vi "Main_Endgame.vi"() -> ()   [LabVIEW 2018]
uses:
  <vilib>/userdefined/High Color/IMAQdx.ctl
  <vilib>/Platform/TimedLoop/XDataNode/timing_clust.ctl
  <vilib>/Platform/TimedLoop/XDataNode/nitl_modes.ctl
  <vilib>/Platform/TimedLoop/XDataNode/wakeup.ctl
  <vilib>/Utility/inputDevices.llb/keyboardAcquire.vi
  <vilib>/Utility/inputDevices.llb/mouseAcquire.vi
  <vilib>/Utility/inputDevices.llb/closeMouse.vi
  <vilib>/Utility/cursorutil.llb/Set Cursor (Icon Pict).vi
  <vilib>/Utility/cursorutil.llb/Set Cursor (Cursor ID).vi
  <vilib>/Platform/TimedLoop/XDataNode/XDataNode.xnode
  <vilib>/Platform/TimedLoop/XDataNode/XDNodeRunTimeDep.lvlib
  <vilib>/vision/driver/NI_Vision_Acquisition_Software.lvlib
panel:
  out "Stop":bool
  in  "default_depth":dbl=120.0
  in  "camera enable":bool
  in  "server port":u16=60006
  in  "listening port":u16=50005
  out "output":dbl[](array[numeric])
  out "beta":dbl
  out "alpha":dbl
  in  "angle_beta_max":dbl=0.2
  in  "angle_beta_min":dbl=-0.7
  in  "angle_alpha_lim":dbl=0.5
  in  "control_region_lim_y":i32=470
  in  "control_region_lim_x":i32=722
  in  "stop_region_lim":i32=90
  in  "UDP enable":bool=TRUE
  in  "Dwell time":dbl=13.0 min=7.0 max=42.0 step=1.0
  out "Boolean 4":bool
  out "Boolean 3":bool
  out "Boolean 2":bool
  out "Boolean":bool
  in  "Cancel Button":bool
  out "Pause_stop":bool
  out "initialized array":i32[](array[numeric])
  out "keys pressed":T1(array[ring])
  out "Local View 2":bool
  out "Image":T2(plugin-control)
  out "Focus":bool
  out "Local View":bool
  out "sd":dbl(graph)
  out "y":i32
  out "x":i32
  out "Global View":bool
  in  "server IP address":string="172.22.11.2"
  out "received data":dbl[](array[numeric])=[0.0, 0.0, 0.0, 0.0, 6000.0]
  out "send data":dbl[](array[numeric])
  out "x_mean":dbl format="%0.2f"
  out "y_mean":dbl format="%0.2f"
  out "y_sd":dbl format="%0.2f"
  out "x_sd":dbl format="%0.2f"
  in  "Stop Button":bool
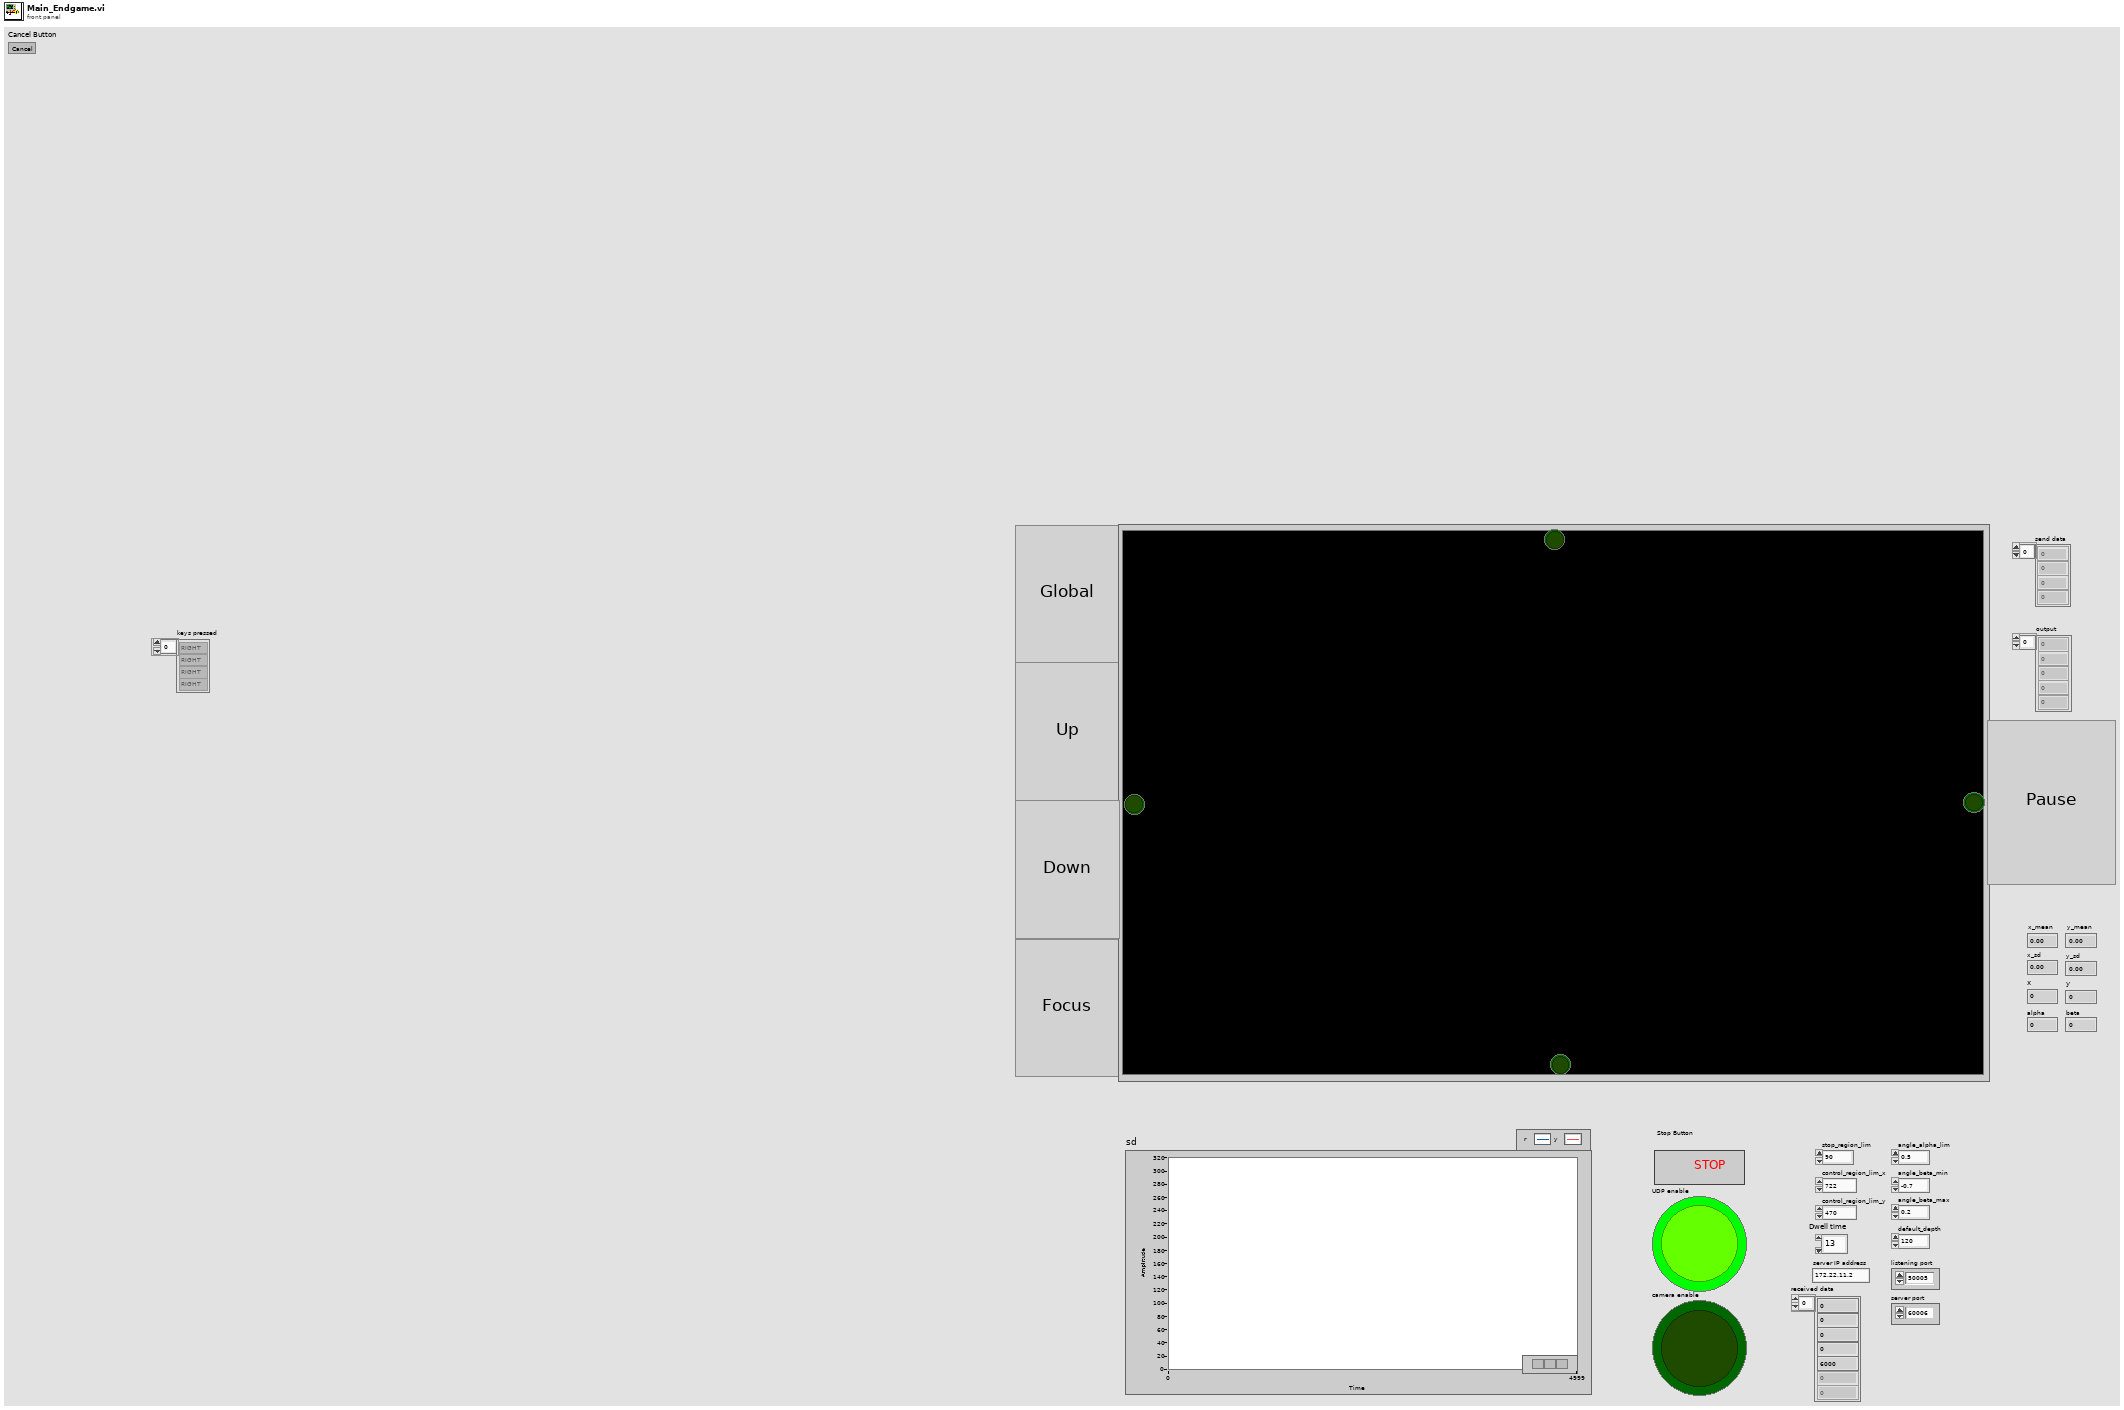
[diagram p1: front panel]
types:
  T1 = enum16{"0", "1", "2", "3", "4", "5", "6", "7", "8", "9", "A", "B", "C", "D", "E", "F", "G", "H", "I", "J", "K", "L", "M", "N", "O", "P", "Q", "R", "S", "T", "U", "V", "W", "X", "Y", "Z", "F1", "F2", "F3", "F4", "F5", "F6", "F7", "F8", "F9", "F10", "F11", "F12", "F13", "F14", "F15", "ADD", "BACK", "BACKSLASH", "CAPITAL", "COMMA", "DECIMAL", "DELETE", "DIVIDE", "DOWN", "END", "EQUALS", "ESCAPE", "GRAVE (`)", "HOME", "INSERT", "LBRACKET", "LCONTROL", "LEFT", "L ALT", "LSHIFT", "LWIN", "MINUS", "MULTIPLY", "NEXT", "NUMLOCK", "NUMPAD_0", "NUMPAD_1", "NUMPAD_2", "NUMPAD_3", "NUMPAD_4", "NUMPAD_5", "NUMPAD_6", "NUMPAD_7", "NUMPAD_8", "NUMPAD_9", "PAUSE", "PERIOD", "PRIOR (PG UP)", "RBRACKET", "RCONTROL", "RETURN", "RIGHT", "R ALT", "RSHIFT", "RWIN", "SCROLL", "SEMICOLON", "SLASH", "SPACE", "SUBTRACT", "TAB", "UP", "ENTER (num pad)", "' (quote)"}[]
  T2 = typedef "IMAQ Image.ctl" = refnum<image>
  T3 = enum16{"0", "1", "2", "3", "4", "5", "6", "7", "8", "9", "A", "B", "C", "D", "E", "F", "G", "H", "I", "J", "K", "L", "M", "N", "O", "P", "Q", "R", "S", "T", "U", "V", "W", "X", "Y", "Z", "F1", "F2", "F3", "F4", "F5", "F6", "F7", "F8", "F9", "F10", "F11", "F12", "F13", "F14", "F15", "ADD", "BACK", "BACKSLASH", "CAPITAL", "COMMA", "DECIMAL", "DELETE", "DIVIDE", "DOWN", "END", "EQUALS", "ESCAPE", "GRAVE (`)", "HOME", "INSERT", "LBRACKET", "LCONTROL", "LEFT", "L ALT", "LSHIFT", "LWIN", "MINUS", "MULTIPLY", "NEXT", "NUMLOCK", "NUMPAD_0", "NUMPAD_1", "NUMPAD_2", "NUMPAD_3", "NUMPAD_4", "NUMPAD_5", "NUMPAD_6", "NUMPAD_7", "NUMPAD_8", "NUMPAD_9", "PAUSE", "PERIOD", "PRIOR (PG UP)", "RBRACKET", "RCONTROL", "RETURN", "RIGHT", "R ALT", "RSHIFT", "RWIN", "SCROLL", "SEMICOLON", "SLASH", "SPACE", "SUBTRACT", "TAB", "UP", "ENTER (num pad)", "' (quote)"}
  T4 = typedef "XDNodeRunTimeDep.lvlib/timing_clust.ctl" = cluster{"Expected End [f-1]":u64, "Actual End [f-1]":u64, "Finished Late? [f-1]":bool, "Expected End [i-1]":u64, "Actual End [i-1]":u64, "Finished Late? [i-1]":bool, "Expected Start [i]":u64, "Actual Start [i]":u64, "Expected Start [f]":u64, "Actual Start [f]":u64, "Source Name":string, "Structure Name":string, "Period":i64, "Deadline":i64, "Offset":i64, "Start":i64, "Priority":i32, "Timeout":i32, "Mode":T5, "Wakeup Reason":T6, "Error":errorcluster, "Source Type":string, "Secondary Source Type":string, "Global End Time":u64, "Global Start Time":u64, "Frame Duration":u64, "Iteration Duration":u64, "Assigned CPU":i32, "I/O Scan Engine Mode":u32}
  T5 = typedef "XDNodeRunTimeDep.lvlib/nitl_modes.ctl" = enum32{"No Change", "Process missed periods, maintain original phase", "Discard missed periods, maintain original phase", "Process missed periods, ignore original phase", "Discard missed periods, ignore original phase"}
  T6 = typedef "XDNodeRunTimeDep.lvlib/wakeup.ctl" = enum32{"Normal", "Aborted", "Asynchronous wakeup", "Timing source error", "Timed loop error", "Timeout"}
  T7 = typedef "LVRectTypeDef.ctl" = cluster{"Left":i16, "Top":i16, "Right":i16, "Bottom":i16}
  T8 = cluster{"Horizontal":i32, "Vertical":i32, "Scrolling":i32}
  T9 = typedef "LVPointTypeDef.ctl" = cluster{"Horizontal":i16, "Vertical":i16}
  T10 = typedef "IMAQdx.ctl" = refnum<k21>
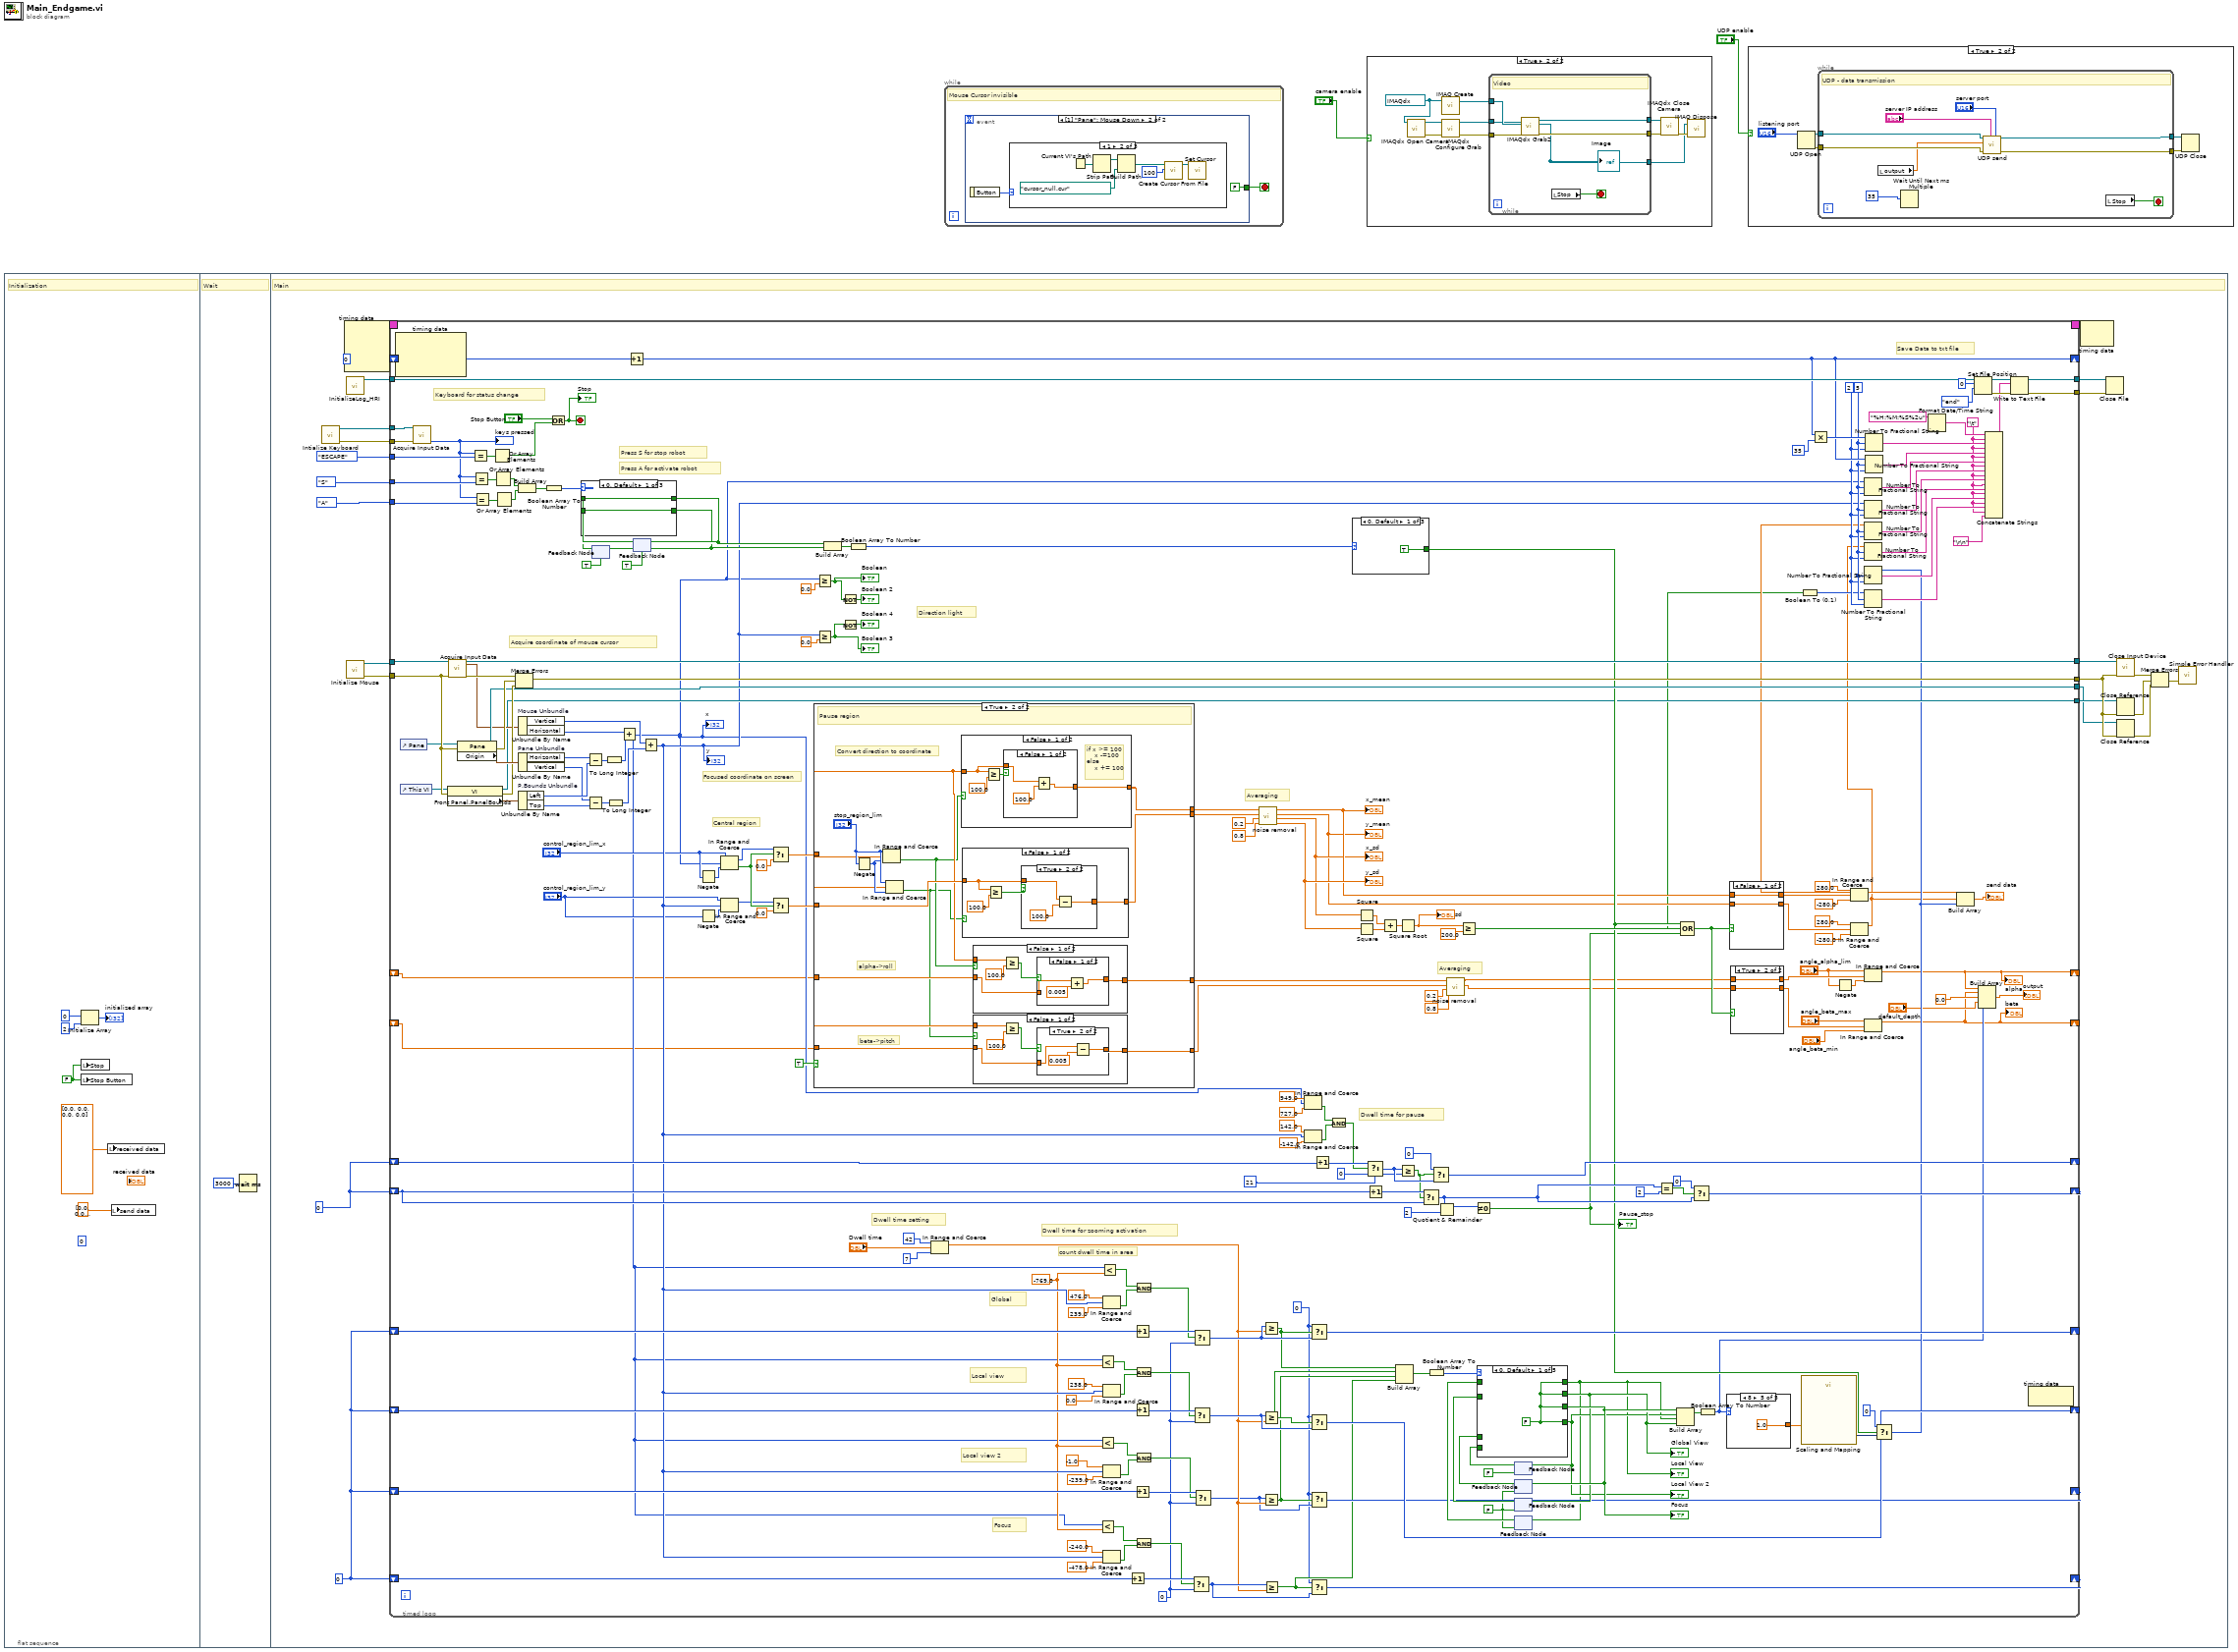
[diagram p0: block diagram]
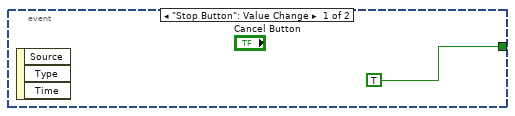
[diagram p4: hidden frame]
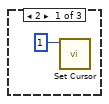
[diagram p5: hidden frame]
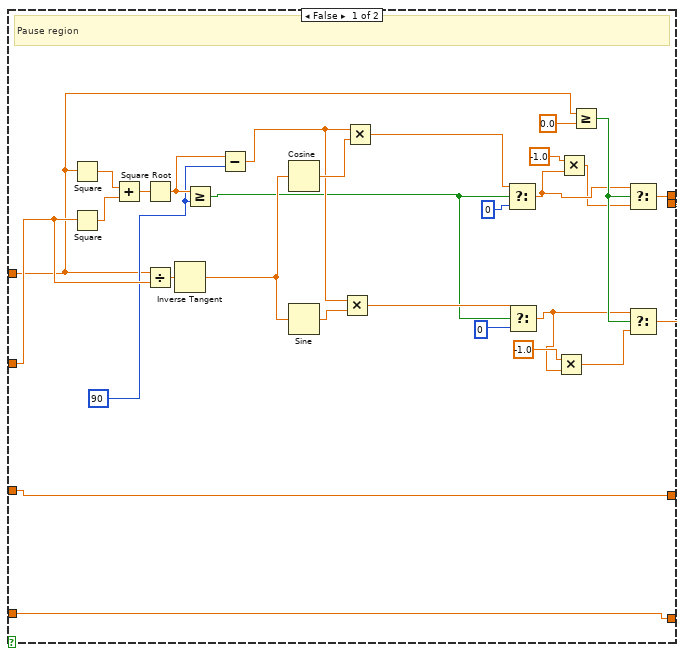
[diagram p8: hidden frame]
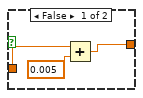
[diagram p9: hidden frame]
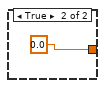
[diagram p10: hidden frame]
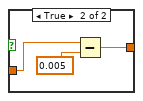
[diagram p11: hidden frame]
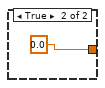
[diagram p12: hidden frame]
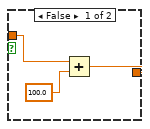
[diagram p13: hidden frame]
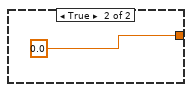
[diagram p14: hidden frame]
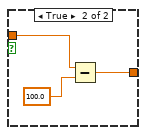
[diagram p15: hidden frame]
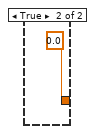
[diagram p16: hidden frame]
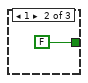
[diagram p17: hidden frame]
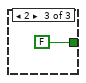
[diagram p18: hidden frame]
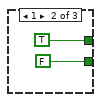
[diagram p19: hidden frame]
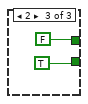
[diagram p20: hidden frame]
diagram:
  n1 = flat-sequence {
    frame #0 {
      (unwired) 0
      w3 = FALSE
      # "Initialization"
      n2 = Initialize Array(0, 2) -> (→"initialized array":i32[])
      n3 = local write "Stop"(w3) -> ()
      n4 = local write "Stop Button"(w3) -> ()
      n5 = local write "received data"(dbl[] [0.0, 0.0, 0.0, 0.0] ("appended array")) -> ()
      n6 = local write "send data"(dbl[] [0.0, 0.0, 0.0, 0.0, 0.0]) -> ()
    }
    frame #1 {
      # "Wait"
      n7 = Wait (ms)(milliseconds to wait=3000) -> ()  [unwired: 1 out]
    }
    frame #2 {
      w12 = 0
      w11 = 0
      # "Main"
      n8 = call <vilib>:"Intialize Keyboard.vi"() -> ("error out"=w19:errorcluster, "device ID"=w20:refnum<k1>)  [unwired: 10 in]
      n9 = node-c288() -> (w32:T4)  [unwired: 4 in]
      n10 = call "InitializeLog_HRI.vi"() -> ("refnum out"=w14:refnum<file>)  [unwired: 11 in]
      n11 = call <vilib>:"Initialize Mouse.vi"() -> ("error out"=w25:errorcluster, "device ID"=w26:refnum<k1>)  [unwired: 10 in]
      n12 = timed-loop {
        timing: w32 -> [_]
        timing-out: [_] -> w31
        shift-right: [w213] -> _
        shift-left: w12 -> [w247]
        shift-right: [w196] -> _
        shift-left: w12 -> [w246]
        tunnel: w26 -> [w232]
        tunnel: w25 -> [w231]
        tunnel: [w228] -> w24
        tunnel: [w227] -> w23
        tunnel: [w226] -> w22
        tunnel: [w116] -> w21
        shift-right: [w215] -> _
        shift-left: w12 -> [w221]
        shift-right: [w194] -> _
        shift-left: w12 -> [w199]
        tunnel: w20 -> [w177]
        tunnel: w19 -> [w176]
        tunnel: T3."ESCAPE" ("keyType 3") -> [w175]
        tunnel: T3."S" ("keyType 3") -> [w174]
        tunnel: T3."A" ("keyType 3") -> [w173]
        tunnel: [w147] -> w15
        tunnel: w14 -> [w146]
        shift-right: [w142] -> _
        shift-left: 0 -> [w145]
        shift-right: [w140] -> _
        shift-left: w11 -> [w141]
        shift-right: [w133] -> _
        shift-left: w11 -> [w138]
        shift-right: [w42] -> _
        shift-left: _ -> [w57]
        shift-right: [w41] -> _
        shift-left: _ -> [w56]
        tunnel: [w47] -> w10
        stop <- w40 stop-if-true
        w118 = 2
        w119 = 5
        w120 = "\t"
        w46 = 0
        w186 = FALSE
        w39 = 0
        w75 = -769.0
        # "count dwell time in area"
        # "Focus"
        # "Local view 2"
        # "Local view"
        # "Global"
        # "Averaging"
        # "Central region"
        # "Focused coordinate on screen"
        # "Averaging"
        # "Keyboard for status change"
        # "Acquire coordinate of mouse cursor"
        # "Direction light"
        # "Dwell time for pause"
        # "Dwell time for zooming activation"
        # "Save Data to txt file"
        # "Dwell time setting"
        # "Press A for activate robot"
        # "Press S for stop robot"
        n13 = node-c288() -> ()  [unwired: 1 in, 4 out]
        n14 = control-ref of="Pane"() -> (w230:refnum<vi>)
        n15 = control-ref of="This VI"() -> (w229:refnum<vi>)
        n16 = call-poly <vilib>:"Acquire Input Data.vi"("device ID"=w177, "error in (no error)"=w176) -> ("keys pressed"=w111:T1)  [unwired: 15 in, 2 out]
        "keys pressed" <- w111
        n17 = property class="VI"(reference=w229, error in=w231) -> (reference out=w116:refnum<vi>, error out=w235:errorcluster, "Front Panel.PanelBounds"=w244:T7)
        n18 = call-poly <vilib>:"Acquire Input Data.vi"("device ID"=w232, "error in (no error)"=w231) -> ("device ID"=w228:refnum<k1>, "axis info"=w225:T8, "error out"=w238:errorcluster)  [unwired: 14 in, 1 out]
        n19 = property class="Pane"(reference=w230, error in=w231) -> (reference out=w226:refnum<vi>, error out=w236:errorcluster, "Origin"=w245:T9)
        n20 = Equal?(x=w111, y=w175) -> (x = y?=w180:bool[])
        n21 = Equal?(x=w111, y=w174) -> (x = y?=w179:bool[])
        n22 = Equal?(x=w111, y=w173) -> (x = y?=w178:bool[])
        n23 = Or Array Elements(Boolean array=w180) -> (logical OR=w104:bool)
        n24 = Or Array Elements(Boolean array=w179) -> (logical OR=w105:bool)
        n25 = Or Array Elements(Boolean array=w178) -> (logical OR=w163:bool)
        n26 = Merge Errors(w238, w236, w235) -> (w227:errorcluster)
        n27 = Unbundle By Name "Mouse Unbundle"(w225) -> ("Vertical"=w224:i32, "Horizontal"=w223:i32)
        n28 = Unbundle By Name "Pane Unbundle"(w245) -> ("Horizontal"=w243:i16, "Vertical"=w241:i16)
        n29 = Unbundle By Name "P.Bounds Unbundle"(w244) -> ("Left"=w242:i16, "Top"=w240:i16)
        n30 = Build Array(w105, w163) -> (w171:bool[])
        n31 = Boolean Array To Number(Boolean array=w171) -> (number=w172:u32)
        n32 = Or(x="Stop Button", y=w104) -> (x .or. y?=w40:bool)
        "Stop" <- w40
        n33 = Subtract(x=w243, y=w242) -> (x-y=w237:i16)
        n34 = Subtract(x=w241, y=w240) -> (x-y=w239:i16)
        n35 = feedback #1(TRUE) -> (w167:bool)
        n36 = To Long Integer(number=w237) -> (32bit integer=w234:i32)
        n37 = To Long Integer(number=w239) -> (32bit integer=w233:i32)
        n38 = Add(x=w223, y=w234) -> (x+y=w60:i32)
        "x" <- w60
        n39 = Increment(x=w145) -> (x+1=w142:i32)
        n40 = feedback #2(TRUE) -> (w168:bool)
        n41 = case shown="0, Default" w172 {
          tunnel: [w356 FALSE TRUE] -> w165
          tunnel: [w357 TRUE FALSE] -> w166
          tunnel: w168 -> [w357 _ _]
          tunnel: w167 -> [w356 _ _]
          frame 0, Default {
          }
          frame 1 {
          }
          frame 2 {
          }
        }
        n42 = feedback-in #1(w165) -> ()
        n43 = feedback-in #2(w166) -> ()
        n44 = Add(x=w224, y=w233) -> (x+y=w79:i32)
        "y" <- w79
        n45 = Negate(x="control_region_lim_x") -> (-x=w64:i32)
        n46 = Negate(x="control_region_lim_y") -> (-x=w62:i32)
        n47 = In Range and Coerce(upper limit="control_region_lim_x", x=w60, lower limit=w64) -> (coerced(x)=w125:i32, In Range?=w126:bool)
        n48 = In Range and Coerce(upper limit="control_region_lim_y", x=w79, lower limit=w62) -> (coerced(x)=w124:i32)  [unwired: 1 out]
        n49 = Select(t=w125, s=w126, f=0.0) -> (s? t:f=w129:dbl)
        n50 = Select(t=w124, s=w126, f=0.0) -> (s? t:f=w127:dbl)
        n51 = case shown="True" TRUE {
          tunnel: w129 -> [w278 w297]
          tunnel: w127 -> [w291 w298]
          tunnel: [w268 w306] -> w107
          tunnel: [w270 w305] -> w106
          tunnel: w57 -> [w267 w302]
          tunnel: [w267 w301] -> w38
          tunnel: w56 -> [w266 w300]
          tunnel: [w266 w299] -> w35
          frame False {
            w287 = 90
            # "Pause region"
            n52 = Square(x=w278) -> (x^2=w292:dbl)
            n53 = Square(x=w291) -> (x^2=w294:dbl)
            n54 = Add(x=w292, y=w294) -> (x+y=w293:dbl)
            n55 = Square Root(x=w293) -> (sqrt(x)=w288:dbl)
            n56 = Divide(x=w278, y=w291) -> (x/y=w286:dbl)
            n57 = Inverse Tangent(1:w286) -> (0:w285:dbl)
            n58 = Greater Or Equal?(x=w288, y=w287) -> (x >= y?=w269:bool)
            n59 = Subtract(x=w288, y=w287) -> (x-y=w281:dbl)
            n60 = Cosine(x=w285) -> (cos(x)=w284:dbl)
            n61 = Sine(x=w285) -> (sin(x)=w282:dbl)
            n62 = Multiply(x=w281, y=w282) -> (x*y=w280:dbl)
            n63 = Multiply(x=w281, y=w284) -> (x*y=w283:dbl)
            n64 = Select(t=w283, s=w269, f=0) -> (s? t:f=w275:dbl)
            n65 = Select(t=w280, s=w269, f=0) -> (s? t:f=w272:dbl)
            n66 = Multiply(x=-1.0, y=w272) -> (x*y=w271:dbl)
            n67 = Multiply(x=-1.0, y=w275) -> (x*y=w274:dbl)
            n68 = Greater Or Equal?(x=w278, y=0.0) -> (x >= y?=w277:bool)
            n69 = Select(t=w275, s=w277, f=w274) -> (s? t:f=w268:dbl)
            n70 = Select(t=w272, s=w277, f=w271) -> (s? t:f=w270:dbl)
          }
          frame True {
            # "beta->pitch"
            # "alpha->roll"
            # "Convert direction to coordinate"
            # "Pause region"
            n71 = Negate(x="stop_region_lim") -> (-x=w303:i32)
            n72 = In Range and Coerce(upper limit="stop_region_lim", x=w297, lower limit=w303) -> (In Range?=w296:bool)  [unwired: 1 out]
            n73 = In Range and Coerce(upper limit="stop_region_lim", x=w298, lower limit=w303) -> (In Range?=w295:bool)  [unwired: 1 out]
            n74 = case shown="False" w296 {
              tunnel: w297 -> [w343 _]
              tunnel: [w342 0.0] -> w306
              frame False {
                # "if x >= 100 \n    x -=100\nelse\n    x += 100"
                n75 = Greater Or Equal?(x=w343, y=100.0) -> (x >= y?=w345:bool)
                n76 = case shown="False" w345 {
                  tunnel: w343 -> [w347 w350]
                  tunnel: [w346 w349] -> w342
                  frame False {
                    n77 = Add(x=w347, y=100.0) -> (x+y=w346:dbl)
                  }
                  frame True {
                    n78 = Subtract(x=w350, y=100.0) -> (x-y=w349:dbl)
                  }
                }
              }
              frame True {
              }
            }
            n79 = case shown="False" w295 {
              tunnel: [w332 0.0] -> w305
              tunnel: w298 -> [w331 _]
              frame False {
                n80 = Greater Or Equal?(x=w331, y=100.0) -> (x >= y?=w334:bool)
                n81 = case shown="True" w334 {
                  tunnel: w331 -> [w336 w339]
                  tunnel: [w335 w338] -> w332
                  frame False {
                    n82 = Add(x=w336, y=100.0) -> (x+y=w335:dbl)
                  }
                  frame True {
                    n83 = Subtract(x=w339, y=100.0) -> (x-y=w338:dbl)
                  }
                }
              }
              frame True {
              }
            }
            n84 = case shown="False" w296 {
              tunnel: w302 -> [w321 _]
              tunnel: [w320 0.0] -> w301
              tunnel: w297 -> [w319 _]
              frame False {
                n85 = Greater Or Equal?(x=w319, y=100.0) -> (x >= y?=w323:bool)
                n86 = case shown="False" w323 {
                  tunnel: w321 -> [w325 w327]
                  tunnel: [w324 w328] -> w320
                  frame False {
                    n87 = Add(x=w325, y=0.005) -> (x+y=w324:dbl)
                  }
                  frame True {
                    n88 = Subtract(x=w327, y=0.005) -> (x-y=w328:dbl)
                  }
                }
              }
              frame True {
              }
            }
            n89 = case shown="False" w295 {
              tunnel: w300 -> [w308 _]
              tunnel: [w309 0.0] -> w299
              tunnel: w298 -> [w307 _]
              frame False {
                n90 = Greater Or Equal?(x=w307, y=100.0) -> (x >= y?=w311:bool)
                n91 = case shown="True" w311 {
                  tunnel: w308 -> [w313 w315]
                  tunnel: [w312 w316] -> w309
                  frame False {
                    n92 = Add(x=w313, y=0.005) -> (x+y=w312:dbl)
                  }
                  frame True {
                    n93 = Subtract(x=w315, y=0.005) -> (x-y=w316:dbl)
                  }
                }
              }
              frame True {
              }
            }
          }
        }
        n94 = Greater Or Equal?(x=w60, y=0.0) -> (x >= y?=w115:bool)
        "Boolean" <- w115
        n95 = Greater Or Equal?(x=w79, y=0.0) -> (x >= y?=w113:bool)
        "Boolean 3" <- w113
        n96 = Build Array(w166, w165) -> (w164:bool[])
        n97 = Not(x=w115) -> (.not. x?=→"Boolean 2":bool)
        n98 = Not(x=w113) -> (.not. x?=→"Boolean 4":bool)
        n99 = Boolean Array To Number(Boolean array=w164) -> (number=w161:u32)
        n100 = In Range and Coerce(upper limit=42, x="Dwell time", lower limit=7) -> (coerced(x)=w103:dbl)  [unwired: 1 out]
        n101 = Less?(x=w60, y=w75) -> (x < y?=w183:bool)
        n102 = Less?(x=w60, y=w75) -> (x < y?=w182:bool)
        n103 = Less?(x=w60, y=w75) -> (x < y?=w181:bool)
        n104 = Less?(x=w60, y=w75) -> (x < y?=w184:bool)
        n105 = In Range and Coerce(upper limit=476.0, x=w79, lower limit=239.0) -> (In Range?=w222:bool)  [unwired: 1 out]
        n106 = In Range and Coerce(upper limit=238.0, x=w79, lower limit=0.0) -> (In Range?=w250:bool)  [unwired: 1 out]
        n107 = In Range and Coerce(upper limit=-1.0, x=w79, lower limit=-239.0) -> (In Range?=w255:bool)  [unwired: 1 out]
        n108 = In Range and Coerce(upper limit=-240.0, x=w79, lower limit=-478.0) -> (In Range?=w202:bool)  [unwired: 1 out]
        n109 = Increment(x=w199) -> (x+1=w204:i32)
        n110 = Increment(x=w221) -> (x+1=w220:i32)
        n111 = Increment(x=w247) -> (x+1=w252:i32)
        n112 = Increment(x=w246) -> (x+1=w257:i32)
        n113 = And(x=w184, y=w222) -> (x .and. y?=w219:bool)
        n114 = And(x=w183, y=w250) -> (x .and. y?=w251:bool)
        n115 = And(x=w182, y=w255) -> (x .and. y?=w256:bool)
        n116 = And(x=w181, y=w202) -> (x .and. y?=w203:bool)
        n117 = Select(t=w204, s=w203, f=w46) -> (s? t:f=w195:i32)
        n118 = Select(t=w220, s=w219, f=w46) -> (s? t:f=w216:i32)
        n119 = Select(t=w252, s=w251, f=w46) -> (s? t:f=w214:i32)
        n120 = Select(t=w257, s=w256, f=w46) -> (s? t:f=w73:i32)
        n121 = call "noise removal.vi"("after14"=0.8, "before14"=0.2, "y"=w106, "x"=w107) -> ("sdy"=w84:dbl, "sdx"=w82:dbl, "newy"=w81:dbl, "newx"=w83:dbl)  [unwired: 4 in]
        "x_mean" <- w83
        "y_mean" <- w81
        "y_sd" <- w84
        "x_sd" <- w82
        n122 = Greater Or Equal?(x=w216, y=w103) -> (x >= y?=w208:bool)
        n123 = Greater Or Equal?(x=w214, y=w103) -> (x >= y?=w74:bool)
        n124 = Greater Or Equal?(x=w73, y=w103) -> (x >= y?=w72:bool)
        n125 = Greater Or Equal?(x=w195, y=w103) -> (x >= y?=w193:bool)
        n126 = In Range and Coerce(upper limit=949.0, x=w60, lower limit=727.0) -> (In Range?=w88:bool)  [unwired: 1 out]
        n127 = In Range and Coerce(upper limit=142.0, x=w79, lower limit=-142.0) -> (In Range?=w100:bool)  [unwired: 1 out]
        n128 = Select(t=w39, s=w208, f=w216) -> (s? t:f=w215:i32)
        n129 = Select(t=w39, s=w74, f=w214) -> (s? t:f=w213:i32)
        n130 = Select(t=w39, s=w72, f=w73) -> (s? t:f=w196:i32)
        n131 = Select(t=w39, s=w193, f=w195) -> (s? t:f=w194:i32)
        n132 = Increment(x=w141) -> (x+1=w99:i32)
        n133 = And(x=w88, y=w100) -> (x .and. y?=w97:bool)
        n134 = case shown="0, Default" w161 {
          tunnel: [TRUE FALSE FALSE] -> w131
          frame 0, Default {
          }
          frame 1 {
          }
          frame 2 {
          }
        }
        n135 = Square(x=w82) -> (x^2=w261:dbl)
        n136 = Square(x=w84) -> (x^2=w260:dbl)
        n137 = Select(t=w99, s=w97, f=0) -> (s? t:f=w95:i32)
        n138 = Increment(x=w138) -> (x+1=w90:i32)
        n139 = Add(x=w261, y=w260) -> (x+y=w259:dbl)
        n140 = Build Array(w208, w74, w72, w193) -> (w218:bool[])
        n141 = Square Root(x=w259) -> (sqrt(x)=w80:dbl)
        "sd" <- w80
        n142 = Greater Or Equal?(x=w95, y=21) -> (x >= y?=w89:bool)
        n143 = Select(t=w90, s=w89, f=w138) -> (s? t:f=w134:i32)
        n144 = Boolean Array To Number(Boolean array=w218) -> (number=w217:u32)
        n145 = Select(t=0, s=w89, f=w95) -> (s? t:f=w140:i32)
        n146 = Quotient & Remainder(x=w134, y=2) -> (x-y*floor(x/y)=w45:i32)  [unwired: 1 out]
        n147 = call "noise removal.vi"("after14"=0.8, "before14"=0.2, "y"=w35, "x"=w38) -> ("newy"=w36:dbl, "newx"=w37:dbl)  [unwired: 4 in, 2 out]
        n148 = Greater Or Equal?(x=w80, y=200.0) -> (x >= y?=w139:bool)
        n149 = Not Equal To 0?(x=w45) -> (x != 0?=w44:bool)
        "Pause_stop" <- w44
        n150 = feedback #3(FALSE) -> (w210:bool)
        n151 = feedback #4(w186) -> (w211:bool)
        n152 = feedback #5(w186) -> (w207:bool)
        n153 = feedback #6(w186) -> (w198:bool)
        n154 = case shown="0, Default" w217 {
          tunnel: [w367 TRUE FALSE w377 w379] -> w205
          tunnel: w211 -> [_ _ _ _ _]
          tunnel: [w367 FALSE TRUE w377 w379] -> w192
          tunnel: w210 -> [_ _ _ _ _]
          tunnel: [w367 FALSE FALSE FALSE TRUE] -> w197
          tunnel: w207 -> [_ _ _ _ _]
          tunnel: [w367 FALSE FALSE TRUE w379] -> w191
          tunnel: w198 -> [_ _ _ _ _]
          frame 0, Default {
            w367 = FALSE
          }
          frame 1 {
          }
          frame 2 {
          }
          frame 4 {
            w377 = FALSE
          }
          frame 8 {
            w379 = FALSE
          }
        }
        "Global View" <- w197
        "Local View" <- w191
        "Focus" <- w205
        "Local View 2" <- w192
        n155 = feedback-in #3(w192) -> ()
        n156 = feedback-in #4(w205) -> ()
        n157 = feedback-in #5(w197) -> ()
        n158 = feedback-in #6(w191) -> ()
        n159 = Equal?(x=w134, y=2) -> (x = y?=w136:bool)
        n160 = Build Array(w205, w192, w191, w197) -> (w209:bool[])
        n161 = Compound Arithmetic op=OR(w131, w139, w44) -> (w43:bool)
        n162 = Select(t=0, s=w136, f=w134) -> (s? t:f=w133:i32)
        n163 = Boolean Array To Number(Boolean array=w209) -> (number=w48:u32)
        n164 = case shown="8" w48 {
          tunnel: [1.0 1.8 1.5 1.2 1.0] -> w206
          frame 0, Default {
          }
          frame 1 {
          }
          frame 2 {
          }
          frame 4 {
          }
          frame 8 {
          }
        }
        n165 = case shown="False" w43 {
          tunnel: [w382 w383] -> w102
          tunnel: [w381 w383] -> w101
          tunnel: w83 -> [w382 _]
          tunnel: w81 -> [w381 _]
          frame False {
          }
          frame True {
            w383 = 0.0
          }
        }
        n166 = case shown="True" w43 {
          tunnel: [w263 w265] -> w59
          tunnel: [w262 w264] -> w58
          tunnel: w37 -> [w263 w265]
          tunnel: w36 -> [w262 w264]
          frame False {
          }
          frame True {
          }
        }
        n167 = Boolean To (0,1)(Boolean=w43) -> (0, 1=w117:i16)
        n168 = call "Scaling and Mapping"("Signals"=w206) -> ("Scaled Signals"=w160:dynamicdata)  [unwired: 9 in, 1 out]
        n169 = Multiply(x=w142, y=35) -> (x*y=w143:i32)
        n170 = Negate(x="angle_alpha_lim") -> (-x=w55:dbl)
        n171 = In Range and Coerce(upper limit=280.0, x=w102, lower limit=-280.0) -> (coerced(x)=w70:dbl)  [unwired: 1 out]
        n172 = In Range and Coerce(upper limit=280.0, x=w101, lower limit=-280.0) -> (coerced(x)=w69:dbl)  [unwired: 1 out]
        n173 = Number To Fractional String(number=w69, width (-)=w119, precision (6)=w118) -> (F-format string=w123:string)  [unwired: 1 in]
        n174 = In Range and Coerce(upper limit="angle_alpha_lim", x=w59, lower limit=w55) -> (coerced(x)=w42:dbl)  [unwired: 1 out]
        "alpha" <- w42
        n175 = In Range and Coerce(upper limit="angle_beta_max", x=w58, lower limit="angle_beta_min") -> (coerced(x)=w41:dbl)  [unwired: 1 out]
        "beta" <- w41
        n176 = Number To Fractional String(number=w60, width (-)=w119, precision (6)=w118) -> (F-format string=w156:string)  [unwired: 1 in]
        n177 = Number To Fractional String(number=w79, width (-)=w119, precision (6)=w118) -> (F-format string=w149:string)  [unwired: 1 in]
        n178 = Number To Fractional String(number=w70, width (-)=w119, precision (6)=w118) -> (F-format string=w148:string)  [unwired: 1 in]
        n179 = Number To Fractional String(number=w117, width (-)=w119, precision (6)=w118) -> (F-format string=w121:string)  [unwired: 1 in]
        n180 = Number To Fractional String(number=w143, width (-)=w119, precision (6)=w118) -> (F-format string=w158:string)  [unwired: 1 in]
        n181 = Number To Fractional String(number=w142, width (-)=w119, precision (6)=w118) -> (F-format string=w157:string)  [unwired: 1 in]
        n182 = Select(t=0, s=w131, f=w160) -> (s? t:f=w71:i32)
        n183 = Number To Fractional String(number=w71, width (-)=w119, precision (6)=w118) -> (F-format string=w122:string)  [unwired: 1 in]
        n184 = Format Date/Time String(time format string (%c)="%H:%M:%S%2u") -> (date/time string=w150:string)  [unwired: 2 in]
        n185 = Build Array(w70, w69, w71) -> (→"send data":dbl[])
        n186 = Set File Position(offset (in bytes) (0)=i64 0, refnum=w146, from (0:start)=enum16{"start", "end", "current"}."end") -> (refnum out=w153:refnum<file>, error out=w159:errorcluster)  [unwired: 1 in]
        n187 = Build Array(w42, w41, 0.0, "default_depth", w48) -> (→"output":dbl[])
        n188 = Concatenate Strings(w150, w120, w158, w120, w157, w120, w156, w120, w149, w120, w148, w120, w123, w120, w122, w120, w121, w120, "\r\n") -> (w152:string)
        n189 = Write to Text File(file (use dialog)=w153, text=w152, error in=w159) -> (refnum out=w147:refnum<file>, error out=w47:errorcluster)  [unwired: 1 in, 1 out]
        n190 = node-c288() -> ()  [unwired: 1 in, 1 out]
      }
      n191 = node-c288(w31) -> ()  [unwired: 1 out]
      n192 = Close File(refnum=w15, error in=w10) -> ()  [unwired: 2 out]
      n193 = call-poly <vilib>:"Close Input Device.vi"("error in (no error)"=w23, "device ID"=w24) -> ("error out"=w30:errorcluster)  [unwired: 8 in]
      n194 = Close Reference(reference=w22, error in (no error)=w23) -> (error out=w29:errorcluster)
      n195 = Close Reference(reference=w21, error in (no error)=w23) -> (error out=w28:errorcluster)
      n196 = Merge Errors(w30, w29, w28) -> (w27:errorcluster)
      n197 = call <vilib>:"Simple Error Handler.vi"("error in (no error)"=w27) -> ()  [unwired: 4 in, 5 out]
    }
  }
  n198 = while {
    stop <- w388 stop-if-true
    # "Mouse Cursor invisible"
    n199 = event shown="[1] \"Pane\": Mouse Down" {
      selector: _ -> [_ _]
      dyn-events: _ -> [_ _]
      timeout: _ -> [_ _]
      tunnel: [TRUE ("stop") FALSE ("stop")] -> w388
      event "Stop Button": Value Change {
        n200 = event-data() -> ()  [unwired: 1 in, 3 out]
      }
      event Mouse Down {
        n201 = event-data() -> ("Button"=w391:u16)  [unwired: 1 in]
        n202 = case shown="1" w391 {
          frame 2 {
            n203 = call-poly <vilib>:"Set Cursor.vi"("icon"=u16 1) -> ()  [unwired: 9 in, 2 out]
          }
          frame 1 {
            n204 = Current VI's Path() -> (path=w396:path)
            n205 = Strip Path(path=w396) -> (stripped path=w394:path)  [unwired: 1 out]
            n206 = Build Path(base path=w394, name or relative path=path "cursor_null.cur" ("cursor file")) -> (appended path=w393:path)
            n207 = call <vilib>:"Create Cursor From File.vi"("cursor resource ID"=i16 100, "cursor file"=w393) -> ("cursor ID"=w398:refnum<k1>)  [unwired: 8 in, 1 out]
            n208 = call-poly <vilib>:"Set Cursor.vi"("cursor ID"=w398) -> ()  [unwired: 9 in, 2 out]
          }
          frame Default {
          }
        }
      }
    }
  }
  n209 = case shown="True" "camera enable" {
    frame False {
    }
    frame True {
      w400 = T10 "cam1" ("Session In")
      n210 = call <vilib>:"IMAQdx Open Camera.vi"("Session In"=w400) -> ("error out"=w402:errorcluster, "Session Out"=w401:T10)  [unwired: 9 in]
      n211 = call "IMAQ Create"("Image Name"=w400) -> ("New Image"=w407:T2)  [unwired: 4 in, 1 out]
      n212 = call <vilib>:"IMAQdx Configure Grab.vi"("error in"=w402, "Session In"=w401) -> ("error out"=w406:errorcluster, "Session Out"=w408:T10)  [unwired: 8 in]
      n213 = while {
        tunnel: w408 -> [w414]
        tunnel: w407 -> [w415]
        tunnel: w406 -> [w413]
        tunnel: [w412] -> w405
        tunnel: [w411] -> w404
        tunnel: [w410] -> w399
        stop <- w409 stop-if-true
        # "Video"
        n214 = call <vilib>:"IMAQdx Grab2.vi"("error in"=w413, "Image In"=w415, "Session In"=w414) -> ("error out"=w411:errorcluster, "Image Out"=w410:T2, "Session Out"=w412:T10)  [unwired: 5 in, 1 out]
        "Image" <- w410
        n215 = local read "Stop"() -> (w409:bool)
      }
      n216 = call <vilib>:"IMAQdx Close Camera.vi"("error in"=w404, "Session In"=w405) -> ("error out"=w403:errorcluster)  [unwired: 9 in]
      n217 = call "IMAQ Dispose"("Image"=w399, "error in (no error)"=w403) -> ()  [unwired: 4 in, 1 out]
    }
  }
  n218 = case shown="True" "UDP enable" {
    frame False {
    }
    frame True {
      n219 = UDP Open(11:"listening port") -> (port=w420:refnum<k16>, 0:w419:errorcluster)  [unwired: 4 in, 1 out]
      n220 = while {
        tunnel: w420 -> [w429]
        tunnel: w419 -> [w428]
        tunnel: [w427] -> w418
        tunnel: [w426] -> w417
        stop <- w421 stop-if-true
        # "UDP - data transmission"
        n221 = local read "output"() -> (w422:dbl[])
        n222 = Wait Until Next ms Multiple(millisecond multiple=35) -> ()  [unwired: 1 out]
        n223 = call "UDP send.vi"("port or service name"="server port", "IP address"="server IP address", "error in"=w428, "Array"=w422, "connection ID in"=w429) -> ("error out"=w426:errorcluster, "connection ID out"=w427:refnum<k16>)  [unwired: 4 in, 1 out]
        n224 = local read "Stop"() -> (w421:bool)
      }
      n225 = UDP Close(connection ID=w418, 8:w417) -> ()  [unwired: 2 out]
    }
  }
